vi "_FPGA_DDS_LUT_initializationVI.vi"() -> (0 "Init Data Out":fxp<+,13,13>[](array[numeric]))   [LabVIEW 2018]
panel:
  # "For Initialization VI requirements and help, please read directions located on Block Diagram."
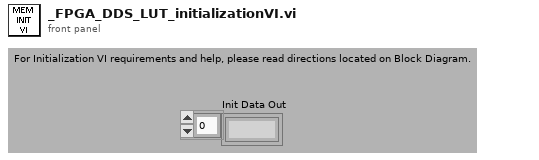
[diagram p1: front panel]
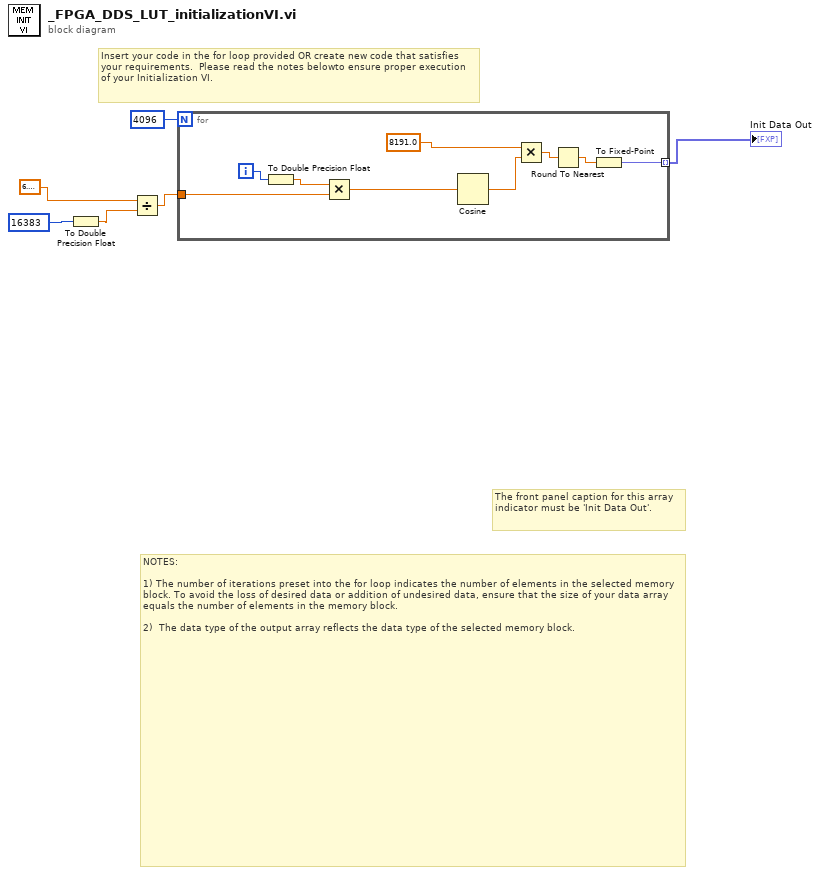
[diagram p0: block diagram]
diagram:
  # "The front panel caption for this array indicator must be 'Init Data Out'."
  # "NOTES:\n\n1) The number of iterations preset into the for loop indicates the number of elements in the selected memory block. To avoid the loss of desired data or addition of undesired data, ensure that the size of your data array equals the number of elements in the memory block.\n\n2)  The data type of the output array reflects the data type of the selected memory block."
  # "Insert your code in the for loop provided OR create new code that satisfies your requirements.  Please read the notes belowto ensure proper execution of your Initialization VI."
  n1 = To Double Precision Float(number=16383) -> (double precision float=w3:dbl)
  n2 = Divide(x=6.283185307179586, y=w3) -> (x/y=w1:dbl)
  n3 = for {
    N: 4096 ("Number of Elements") -> [_]
    tunnel: [w11] -> w5 mode=indexing
    tunnel: w1 -> [w13]
    i -> [w15]
    n4 = To Double Precision Float(number=w15) -> (double precision float=w14:dbl)
    n5 = Multiply(x=w14, y=w13) -> (x*y=w12:dbl)
    n6 = Cosine(x=w12) -> (cos(x)=w10:dbl)
    n7 = Multiply(x=sgl 8191.0, y=w10) -> (x*y=w7:dbl)
    n8 = Round To Nearest(number=w7) -> (nearest integer value=w8:dbl)
    n9 = To Fixed-Point(number=w8) -> (fixed-point=w11:fxp<+,13,13>)  [unwired: 1 in]
  }
  "Init Data Out" <- w5
